vi "Test Program Logging Create Log.vi"(8 "error in":errorcluster, 11 "File Name":string="Test Program Log File") -> (0 "error out":errorcluster, 3 "refnum out":refnum<file>)   [LabVIEW 2018, in "Support Library.lvlib"]
uses:
  support/Support Library.lvlib
  <vilib>/Utility/sysdir.llb/System Directory Type.ctl
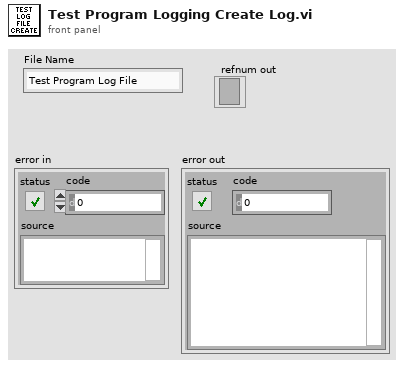
[diagram p1: front panel]
types:
  T1 = typedef "System Directory Type.ctl" = i32
  T2 = enum16{"open", "replace", "create", "open or create", "replace or create", "replace or create with confirmation"}
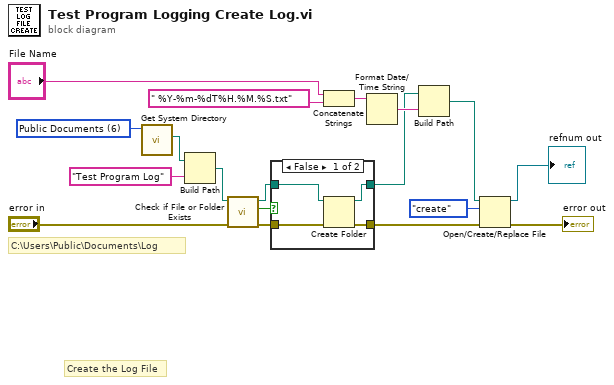
[diagram p0: block diagram]
diagram:
  w17 = T1 6 items=["User Home"=0, "User Desktop"=1, "User Documents"=2, "User Application Data"=3, "User Preferences"=4, "User Temporary"=5, "Public Documents"=6, "Public Application Data"=7, "Public Preferences"=8, "Public Cache"=13, "System Core Libraries"=9, "System Installed Libraries"=10, "Application Files"=11, "Boot Volume Root"=12] ("system directory type")
  # "Create the Log File"
  # "C:\\Users\\Public\\Documents\\Log"
  n1 = call <vilib>:"Get System Directory.vi"("system directory type"=w17) -> ("system directory"=w12:path)  [unwired: 10 in]
  n2 = Build Path(base path=w12, name or relative path="Test Program Log") -> (appended path=w5:path)
  n3 = call <vilib>:"Check if File or Folder Exists.vi"("error in (no error)"="error in", "path"=w5) -> ("error out"=w8:errorcluster, "file or folder exists?"=w7:bool, "dup path"=w6:path)  [unwired: 7 in]
  n4 = case shown="False" w7 {
    tunnel: w6 -> [w22 w24]
    tunnel: w8 -> [w21 w23]
    tunnel: [w20 w24] -> w4
    tunnel: [w19 w23] -> w2
    frame False {
      n5 = Create Folder(path (use dialog)=w22, error in=w21) -> (created path=w20:path, error out=w19:errorcluster)  [unwired: 1 in, 1 out]
    }
    frame True {
    }
  }
  n6 = Concatenate Strings("File Name", " %Y-%m-%dT%H.%M.%S.txt" ("time format string (%c)")) -> (w13:string)
  n7 = Format Date/Time String(time format string (%c)=w13) -> (date/time string=w16:string)  [unwired: 2 in]
  n8 = Build Path(base path=w4, name or relative path=w16) -> (appended path=w14:path)
  n9 = Open/Create/Replace File(file path (use dialog)=w14, error in=w2, operation (0:open)=T2."create") -> (refnum out=→"refnum out":refnum<file>, error out=→"error out":errorcluster)  [unwired: 3 in, 1 out]
